vi "close.vi"(8 "error in (no error)":errorcluster, 11 "CamaraSettings in":refnum<class "CamaraSettings.lvclass">) -> (0 "error out":errorcluster, 3 "CamaraSettings out":refnum<class "CamaraSettings.lvclass">)   [LabVIEW 2011, in "Tools.lvlib" / "Settings.lvlib" / "CamaraSettings.lvclass"]
uses:
  CamaraSettings.lvclass
  CamaraSettings.lvclass/CamaraSettings.ctl
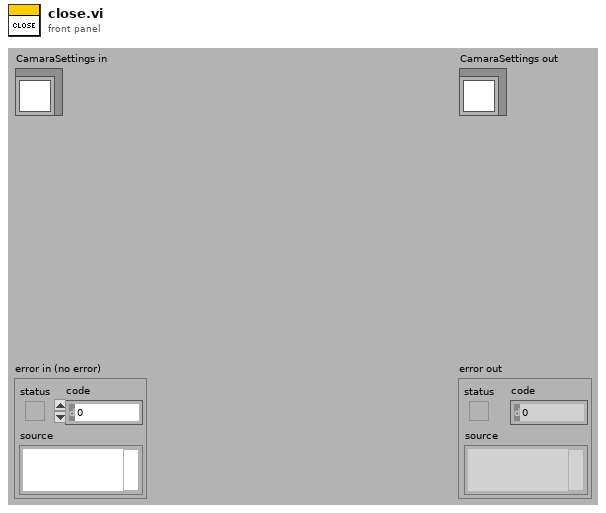
[diagram p1: front panel]
types:
  T1 = enum32{"Bad", "Idle", "Run top level", "Running"}
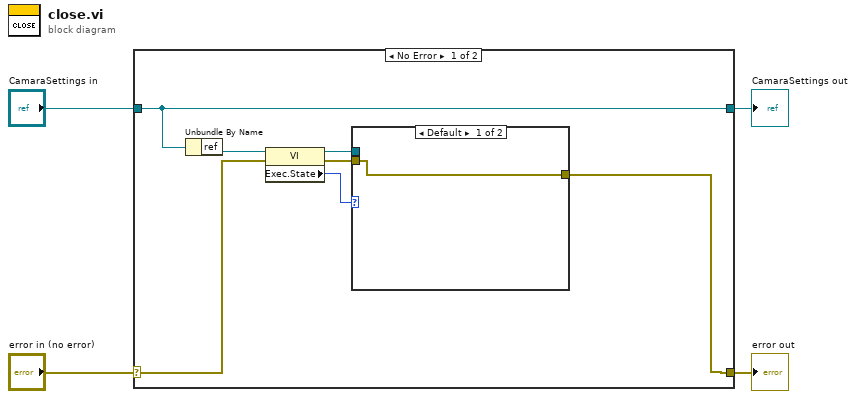
[diagram p0: block diagram]
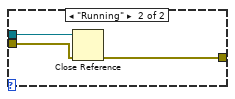
[diagram p2: hidden frame]
diagram:
  n1 = case shown="No Error" "error in (no error)" {
    selector: "error in (no error)" -> [w6 w17]
    tunnel: [w5 w17] -> w3
    tunnel: [w11 w16] -> w1
    tunnel: "CamaraSettings in" -> [w11 w16]
    frame No Error {
      n2 = Unbundle By Name(w11) -> ("ref"=w10:refnum<vi>)
      n3 = property class="VI"(reference=w10, error in=w6) -> (reference out=w8:refnum<vi>, error out=w7:errorcluster, "Exec.State"=w9:T1)
      n4 = case shown="Default" w9 {
        tunnel: w8 -> [_ w15]
        tunnel: w7 -> [w12 w14]
        tunnel: [w12 w13] -> w5
        frame Default {
        }
        frame "Running" {
          n5 = Close Reference(reference=w15, error in (no error)=w14) -> (error out=w13:errorcluster)
        }
      }
    }
    frame Error {
    }
  }
  "error out" <- w3
  "CamaraSettings out" <- w1
